vi "GetWindowTitleBarVisible.vi"(8 "error in (no error)":errorcluster, 11 "WindowFrame in":refnum<class "WindowFrame.lvclass">) -> (0 "error out":errorcluster, 2 "Title Bar Visible":bool, 3 "WindowFrame out":refnum<class "WindowFrame.lvclass">)   [LabVIEW 2021, in "WindowFrame.lvlib" / "WindowFrame.lvclass"]
uses:
  WindowFrame.lvclass
  Action.ctl
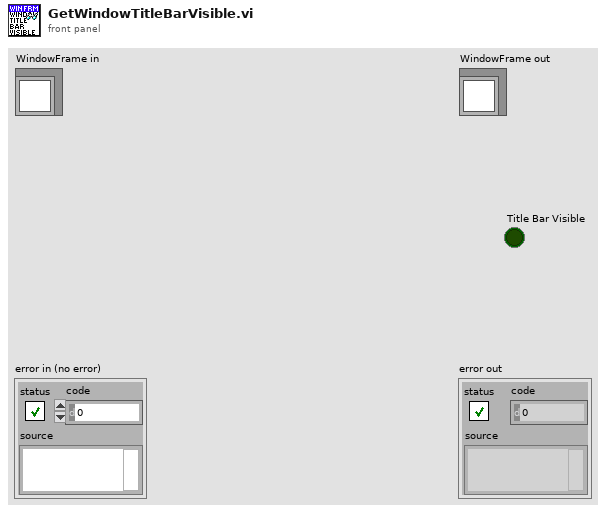
[diagram p1: front panel]
types:
  T1 = typedef "WindowFrame.lvlib/WindowFrame.lvclass/Action.ctl" = enum16{"Set Allow Runtime PopUp", "Set Behavior", "Set Closable", "Set Custom Title", "Set Highlight Return Button", "Set Is Frontmost", "Set Minimizable", "Set Minimum Size", "Set Monitor", "Set Resizable", "Set Panel Bounds", "Set Run VI Transparently", "Set Show Menu Bar", "Set State", "Set Title", "Set Title Bar Colors", "Set Title Bar Visible", "Set Transparancy", "Set Window Bounds", "Get Allow Runtime PopUp", "Get Behavior", "Get Closable", "Get Custom Title", "Get Highlight Return Button", "Get Is Frontmost", "Get Minimizable", "Get Minimum Size", "Get Monitor", "Get Panel Bounds", "Get Resizable", "Get Run VI Transparently", "Get Show Menu Bar", "Get State", "Get Title", "Get Title Bar Colors", "Get Title Bar Visible", "Get Transparancy", "Get Window Bounds", "--", "Center", "Close", "Open", "Run-Time Position:Centered", "Run-Time Position:Custom", "Run-Time Position:Get Position", "Run-Time Position:Maximized", "Run-Time Position:Minimized", "Run-Time Position:Unchanged", "---", "Insert VI", "Remove VI", "Insert VI Index", "Remove VI Index", "Exit"}
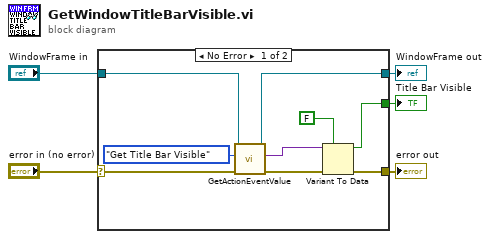
[diagram p0: block diagram]
diagram:
  n1 = case shown="No Error" "error in (no error)" {
    selector: "error in (no error)" -> [w8 w16]
    tunnel: [w9 w16] -> w4
    tunnel: [w6 w15] -> w2
    tunnel: "WindowFrame in" -> [w7 w15]
    tunnel: [w10 _] -> w1
    frame No Error {
      n2 = call "GetActionEventValue.vi"("error in (no error)"=w8, "Action"=Action."Get Title Bar Visible", "WindowFrame in"=w7) -> ("error out"=w13:errorcluster, "Variant"=w12:variant, "WindowFrame out"=w6:refnum<class "WindowFrame.lvclass">)  [unwired: 6 in]
      n3 = Variant To Data(error in=w13, type=FALSE, Variant=w12) -> (data=w10:bool, error out=w9:errorcluster)
    }
    frame Error {
    }
  }
  "error out" <- w4
  "WindowFrame out" <- w2
  "Title Bar Visible" <- w1
